vi "SetGraphLegend.vi"(4 "error in (no error)":errorcluster, 5 "GraphIndex":T2, 6 "ConfigTotale":T3, 7 "ClusterRefGraphs":T1) -> (0 "error out":errorcluster)   [LabVIEW 2017]
uses:
  DefDeType/ConfigTotale.ctl
  DefDeType/VoltageChannels.ctl
  DefDeType/WBridgeChannels.ctl
  DefDeType/Configuration.ctl
panel:
  out "sortie d'erreur 2":errorcluster caption="sortie d'erreur"
  out "sortie d'erreur":errorcluster
  out "entier 32 bits non signé":u32
  out "Array 2":string[](array[string])
  out "Array":string[](array[string])
  out "appended array":string[](array[string])
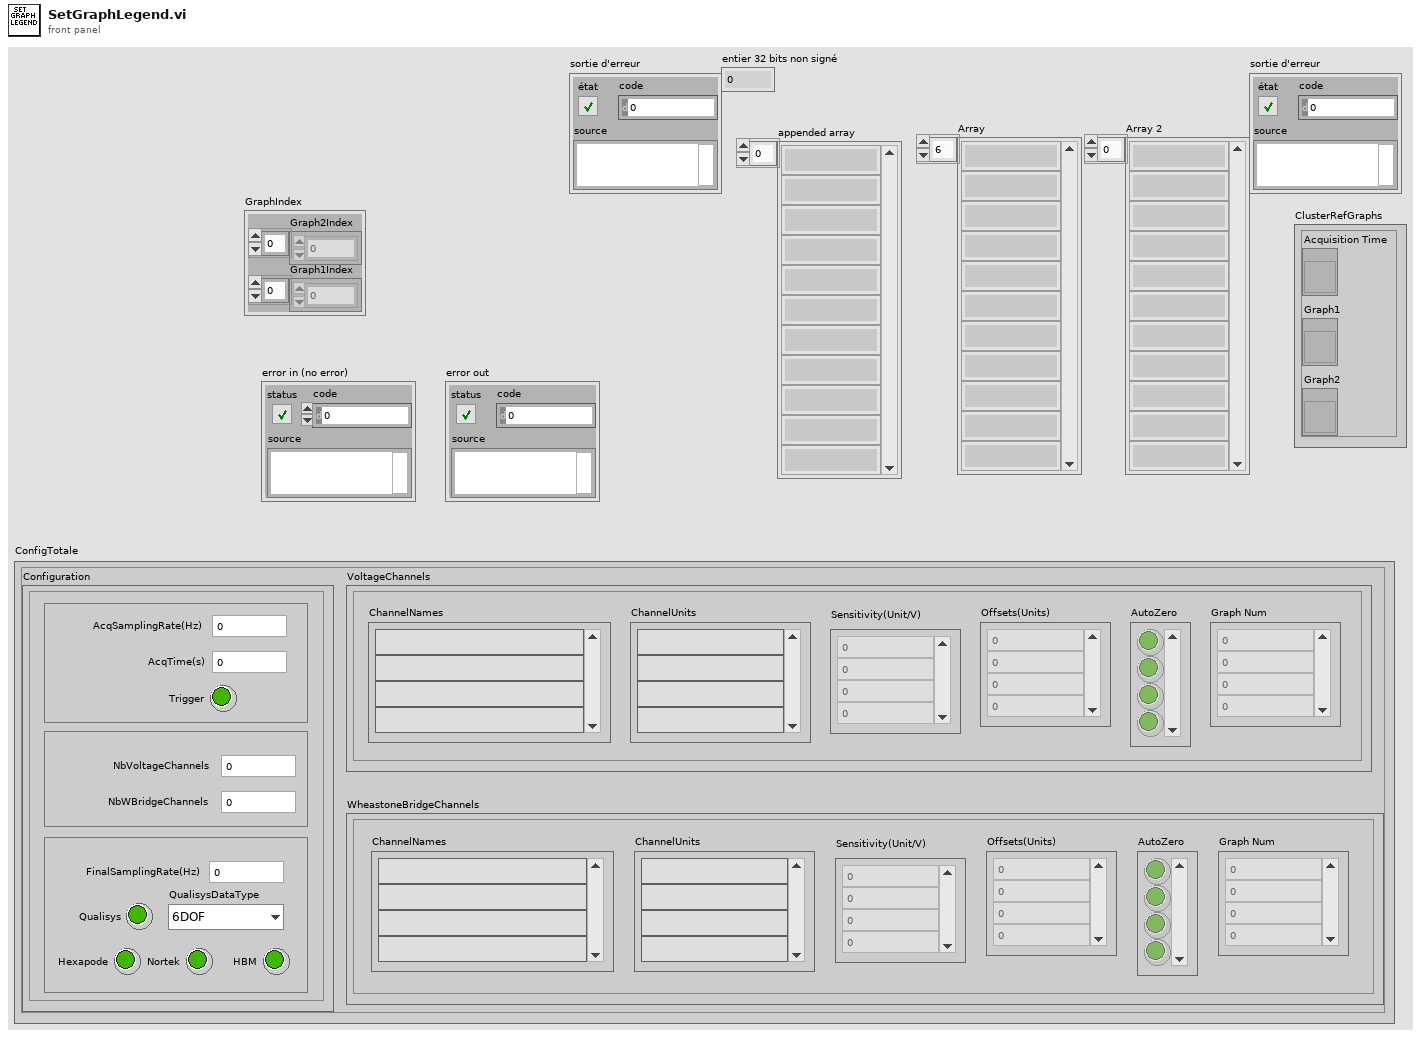
[diagram p1: front panel]
types:
  T1 = cluster{"Acquisition Time":refnum<vi>, "Graph1":refnum<vi>, "Graph2":refnum<vi>}
  T2 = cluster{"Graph2Index":i32[], "Graph1Index":i32[]}
  T3 = typedef "ConfigTotale.ctl" = cluster{"VoltageChannels":T4, "WheastoneBridgeChannels":T5, "Configuration":T6}
  T4 = typedef "VoltageChannels.ctl" = cluster{"ChannelNames":string[], "Sensitivity(Unit/V)":dbl[], "AutoZero":bool[], "ChannelUnits":string[], "Offsets(Units)":dbl[], "Graph Num":u8[]}
  T5 = typedef "WBridgeChannels.ctl" = cluster{"ChannelNames":string[], "Sensitivity(Unit/V)":dbl[], "AutoZero":bool[], "ChannelUnits":string[], "Offsets(Units)":dbl[], "Graph Num":u8[]}
  T6 = typedef "Configuration.ctl" = cluster{"AcqSamplingRate(Hz)":u32, "AcqTime(s)":u32, "Trigger":bool, "NbVoltageChannels":u32, "NbWBridgeChannels":u32, "Qualisys":bool, "Hexapode":bool, "FinalSamplingRate(Hz)":u32, "QualisysDataType":enum16{"6DOF", "3DTracking", "6DOF + 3D"}, "Nortek":bool, "HBM":bool}
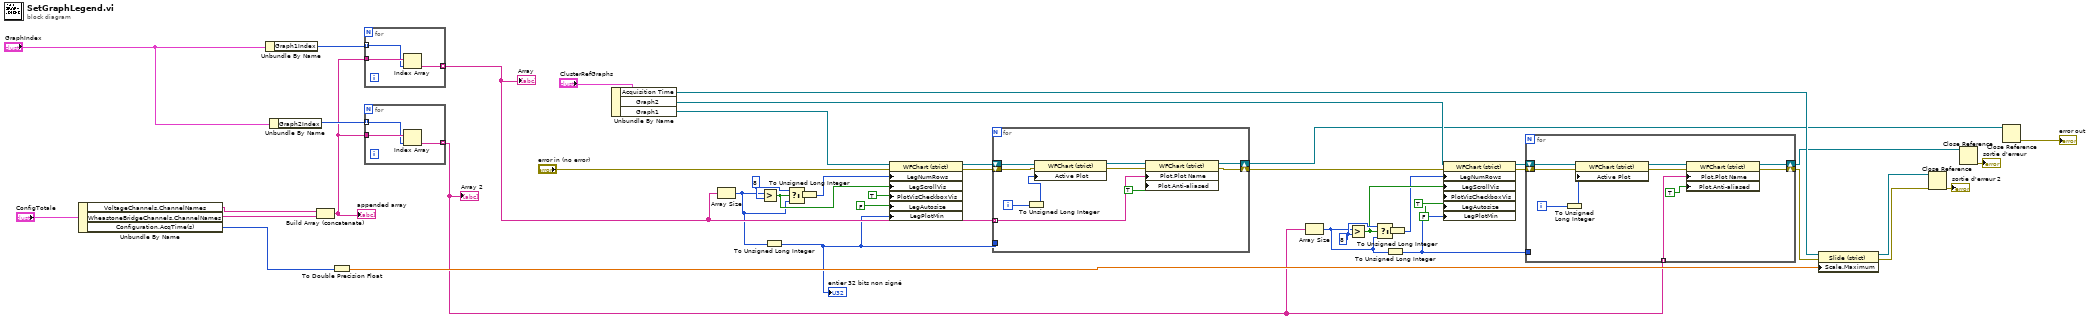
[diagram p0: block diagram]
diagram:
  w21 = 8 ("y")
  w24 = 8 ("y")
  n1 = Unbundle By Name("ConfigTotale") -> ("VoltageChannels.ChannelNames"=w36:string[], "WheastoneBridgeChannels.ChannelNames"=w35:string[], "Configuration.AcqTime(s)"=w30:u32)
  n2 = Unbundle By Name("GraphIndex") -> ("Graph1Index"=w34:i32[])
  n3 = Unbundle By Name("GraphIndex") -> ("Graph2Index"=w32:i32[])
  n4 = Build Array (concatenate)(w36, w35) -> (w31:string[])
  "appended array" <- w31
  n5 = To Double Precision Float(number=w30) -> (double precision float=w45:dbl)
  n6 = for {
    tunnel: w34 -> [w47] mode=indexing
    tunnel: w31 -> [w48]
    tunnel: [w46] -> w29 mode=indexing
    n7 = Index Array(array=w48, index=w47) -> (element=w46:string)
  }
  "Array" <- w29
  n8 = for {
    tunnel: w32 -> [w50] mode=indexing
    tunnel: w31 -> [w51]
    tunnel: [w49] -> w20 mode=indexing
    n9 = Index Array(array=w51, index=w50) -> (element=w49:string)
  }
  "Array 2" <- w20
  n10 = Unbundle By Name("ClusterRefGraphs") -> ("Acquisition Time"=w25:refnum<vi>, "Graph2"=w26:refnum<vi>, "Graph1"=w27:refnum<vi>)
  n11 = Array Size(array=w29) -> (size(s)=w6:i32)
  n12 = Greater?(x=w6, y=w24) -> (0:w8:bool)
  n13 = To Unsigned Long Integer(number=w6) -> (unsigned 32bit integer=w1:u32)
  "entier 32 bits non signé" <- w1
  n14 = Select(t=w24, s=w8, f=w6) -> (s? t:f=w23:i32)
  n15 = To Unsigned Long Integer(number=w23) -> (unsigned 32bit integer=w9:u32)
  n16 = property class="WFChart (strict)"(reference=w27, error in="error in (no error)", "LegNumRows"=w9, "LegScrollVis"=w8, "PlotVisCheckboxVis"=TRUE ("Légende:Case de visibilité du tracé visible"), "LegAutosize"=FALSE ("Légende:Redimensionnement automatique"), "LegPlotMin"=w1) -> (reference out=w43:refnum<vi>, error out=w42:errorcluster)
  n17 = for {
    shift-right: [w57] -> w39
    shift-left: w42 -> [w60]
    tunnel: w29 -> [w52] mode=indexing
    tunnel: w1 -> [_]
    shift-right: [w56] -> w10
    shift-left: w43 -> [w61]
    i -> [w54]
    n18 = To Unsigned Long Integer(number=w54) -> (unsigned 32bit integer=w55:u32)
    n19 = property class="WFChart (strict)"(reference=w61, error in=w60, "Active Plot"=w55) -> (reference out=w58:refnum<vi>, error out=w59:errorcluster)
    n20 = property class="WFChart (strict)"(reference=w58, error in=w59, "Plot.Plot Name"=w52, "Plot.Anti-aliased"=TRUE ("Tracé.Visible")) -> (reference out=w56:refnum<vi>, error out=w57:errorcluster)
  }
  n21 = Array Size(array=w20) -> (size(s)=w5:i32)
  n22 = Greater?(x=w5, y=w21) -> (0:w19:bool)
  n23 = Select(t=w21, s=w19, f=w5) -> (s? t:f=w22:i32)
  n24 = To Unsigned Long Integer(number=w5) -> (unsigned 32bit integer=w2:u32)
  n25 = To Unsigned Long Integer(number=w22) -> (unsigned 32bit integer=w7:u32)
  n26 = property class="WFChart (strict)"(reference=w26, error in=w39, "LegNumRows"=w7, "LegScrollVis"=w19, "PlotVisCheckboxVis"=TRUE ("Légende:Case de visibilité du tracé visible"), "LegAutosize"=FALSE ("Légende:Redimensionnement automatique"), "LegPlotMin"=w2) -> (reference out=w40:refnum<vi>, error out=w41:errorcluster)
  n27 = for {
    shift-right: [w67] -> w38
    shift-left: w41 -> [w70]
    tunnel: w20 -> [w63] mode=indexing
    tunnel: w2 -> [_]
    shift-right: [w66] -> w11
    shift-left: w40 -> [w71]
    i -> [w65]
    n28 = To Unsigned Long Integer(number=w65) -> (unsigned 32bit integer=w64:u32)
    n29 = property class="WFChart (strict)"(reference=w71, error in=w70, "Active Plot"=w64) -> (reference out=w68:refnum<vi>, error out=w69:errorcluster)
    n30 = property class="WFChart (strict)"(reference=w68, error in=w69, "Plot.Plot Name"=w63, "Plot.Anti-aliased"=TRUE ("Légende:Case de visibilité du tracé visible")) -> (reference out=w66:refnum<vi>, error out=w67:errorcluster)
  }
  n31 = property class="Slide (strict)"(reference=w25, error in=w38, "Scale.Maximum"=w45) -> (reference out=w12:refnum<vi>, error out=w14:errorcluster)
  n32 = Close Reference(reference=w12, error in (no error)=w14) -> (error out=→"sortie d'erreur 2":errorcluster)
  n33 = Close Reference(reference=w11) -> (error out=→"sortie d'erreur":errorcluster)  [unwired: 1 in]
  n34 = Close Reference(reference=w10) -> (error out=→"error out":errorcluster)  [unwired: 1 in]
